vi "IntegerValueChange.vi"(8 "error in (no error)":errorcluster, 10 "NewVal":i32, 11 "View in":refnum<class "View.lvclass">) -> (0 "error out":errorcluster, 3 "View out":refnum<class "View.lvclass">)   [LabVIEW 2020, in "View.lvclass"]
uses:
  View.lvclass
  View.lvclass/View.ctl
  Controller/Controller.lvclass
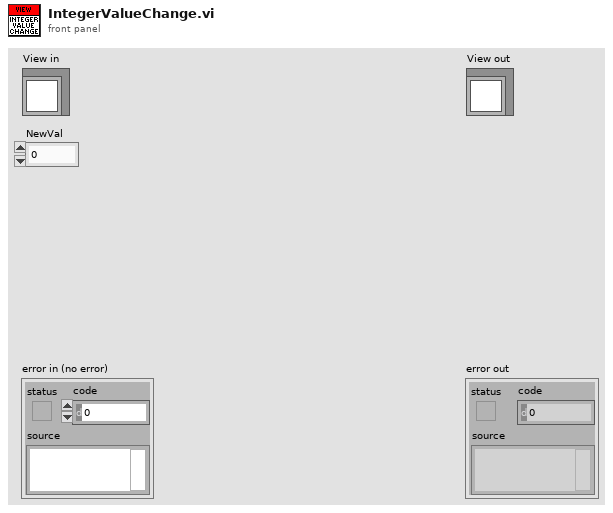
[diagram p1: front panel]
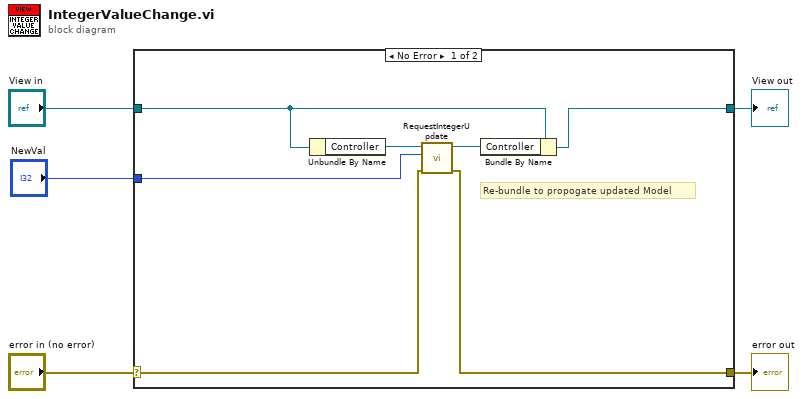
[diagram p0: block diagram]
diagram:
  n1 = case shown="No Error" "error in (no error)" {
    selector: "error in (no error)" -> [w10 w14]
    tunnel: [w9 w14] -> w4
    tunnel: [w6 w13] -> w2
    tunnel: "View in" -> [w7 w13]
    tunnel: "NewVal" -> [w11 _]
    frame No Error {
      # "Re-bundle to propogate updated Model"
      n2 = Unbundle By Name(w7) -> ("Controller"=w12:refnum<class "Controller.lvclass">)
      n3 = call "RequestIntegerUpdate.vi"("error in (no error)"=w10, "NewVal"=w11, "Controller in"=w12) -> ("error out"=w9:errorcluster, "Controller out"=w8:refnum<class "Controller.lvclass">)  [unwired: 7 in]
      n4 = Bundle By Name(cluster=w7, "Controller"=w8) -> (w6:refnum<class "View.lvclass">)
    }
    frame Error {
    }
  }
  "error out" <- w4
  "View out" <- w2
